vi "Get XML Path.vi"(8 "error in (no error)":errorcluster, 11 "RIO Target in":refnum<class "RIO Target.lvclass">) -> (0 "error out":errorcluster, 2 "XML Path":path, 3 "RIO Target out":refnum<class "RIO Target.lvclass">)   [LabVIEW 2014, in "RIO Target.lvclass"]
uses:
  RIO Target.lvclass
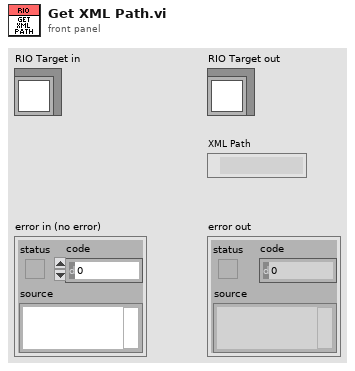
[diagram p1: front panel]
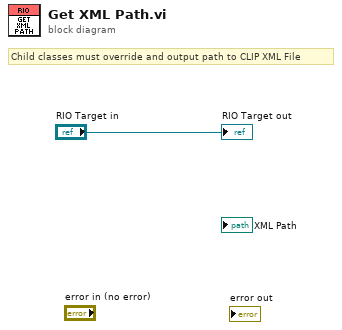
[diagram p0: block diagram]
diagram:
  # "Child classes must override and output path to CLIP XML File"
  "RIO Target out" <- "RIO Target in"
